vi "5_inputs_or_gate.vi"(0 "x":bool, 1 "y":bool, 2 "z":bool, 3 "p":bool, 4 "m":bool) -> (5 "o3":bool)   [LabVIEW 2015]
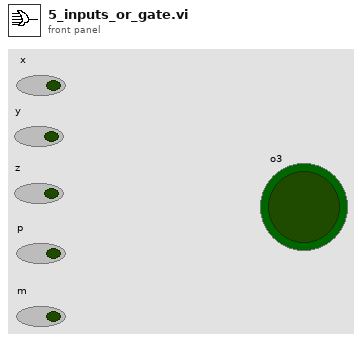
[diagram p1: front panel]
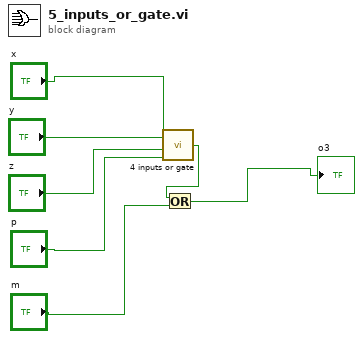
[diagram p0: block diagram]
diagram:
  n1 = call "4 inputs or gate.vi"("p"="p", "z"="z", "y"="y", "x"="x") -> ("o2"=w7:bool)
  n2 = Or(x=w7, y="m") -> (x .or. y?=→"o3":bool)
